vi "Continuous PDF.vi"   [LabVIEW 2020, in "NI_Gmath.lvlib"]
doc: "Computes the continuous probability density function (PDF) of various distributions. You must manually select the polymorphic instance to use."
uses:
  <vilib>/gmath/NI_Gmath.lvlib
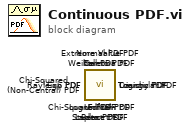
[diagram p0: block diagram]
diagram:
  n1 = call <vilib>:"Lognormal PDF.vi"() -> ()  [unwired: 10 in, 2 out]
  n2 = call <vilib>:"Pareto PDF.vi"() -> ()  [unwired: 10 in, 2 out]
  n3 = call <vilib>:"Chi-Squared (Non-Central) PDF.vi"() -> ()  [unwired: 10 in, 2 out]
  n4 = call <vilib>:"Logistic PDF.vi"() -> ()  [unwired: 10 in, 2 out]
  n5 = call <vilib>:"Laplace PDF.vi"() -> ()  [unwired: 10 in, 2 out]
  n6 = call <vilib>:"Extreme Value PDF.vi"() -> ()  [unwired: 10 in, 2 out]
  n7 = call <vilib>:"Weibull PDF.vi"() -> ()  [unwired: 10 in, 2 out]
  n8 = call <vilib>:"Uniform PDF.vi"() -> ()  [unwired: 10 in, 2 out]
  n9 = call <vilib>:"Triangular PDF.vi"() -> ()  [unwired: 10 in, 2 out]
  n10 = call <vilib>:"Student t PDF.vi"() -> ()  [unwired: 10 in, 2 out]
  n11 = call <vilib>:"Rayleigh PDF.vi"() -> ()  [unwired: 10 in, 2 out]
  n12 = call <vilib>:"Normal PDF.vi"() -> ()  [unwired: 10 in, 2 out]
  n13 = call <vilib>:"Gamma PDF.vi"() -> ()  [unwired: 10 in, 2 out]
  n14 = call <vilib>:"F PDF.vi"() -> ()  [unwired: 10 in, 2 out]
  n15 = call <vilib>:"Exp PDF.vi"() -> ()  [unwired: 10 in, 2 out]
  n16 = call <vilib>:"Chi-Squared PDF.vi"() -> ()  [unwired: 10 in, 2 out]
  n17 = call <vilib>:"Cauchy PDF.vi"() -> ()  [unwired: 10 in, 2 out]
  n18 = call <vilib>:"Beta PDF.vi"() -> ()  [unwired: 10 in, 2 out]
